vi "test Buffer String to Display String.vi"(8 "error in (no error)":errorcluster, 11 "TestCase in":refnum<class "Buffer Tests.lvclass">=refnum) -> (0 "error out":errorcluster, 3 "TestCase out":refnum<class "Buffer Tests.lvclass">)   [LabVIEW 2021, in "Buffer Tests.lvclass"]
uses:
  Buffer Tests.lvclass
  DSF Core.lvlib
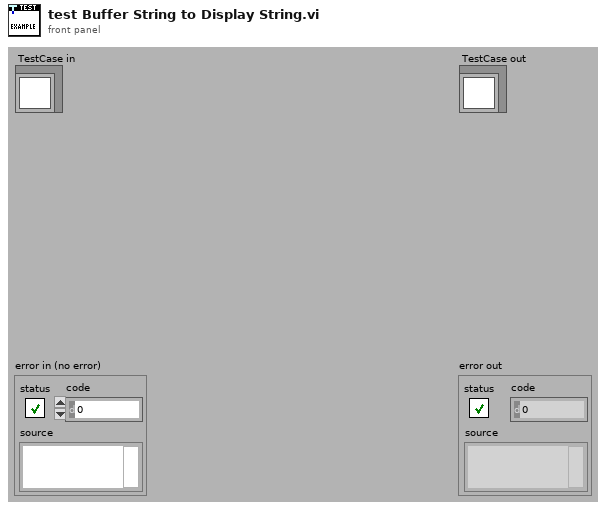
[diagram p1: front panel]
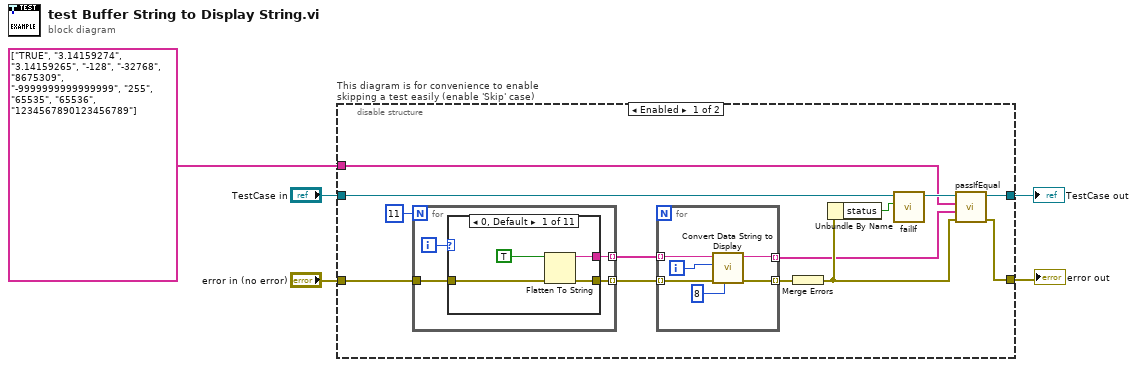
[diagram p0: block diagram]
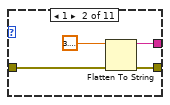
[diagram p2: hidden frame]
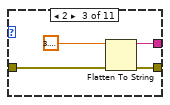
[diagram p3: hidden frame]
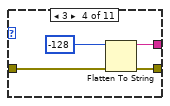
[diagram p4: hidden frame]
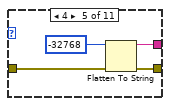
[diagram p5: hidden frame]
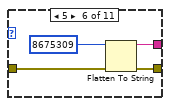
[diagram p6: hidden frame]
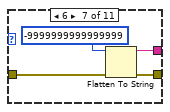
[diagram p7: hidden frame]
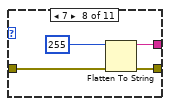
[diagram p8: hidden frame]
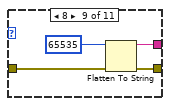
[diagram p9: hidden frame]
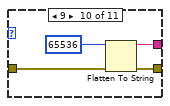
[diagram p10: hidden frame]
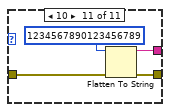
[diagram p11: hidden frame]
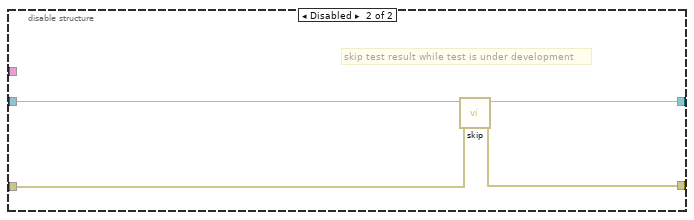
[diagram p12: hidden frame]
diagram:
  n1 = disable-structure "This diagram is for convenience to enable skipping a test easily (enable 'Skip' case)" shown="Enabled" {
    disable-tunnel: "TestCase in" -> [w12 w76]
    disable-tunnel: [w18 w74] -> w2
    disable-tunnel: [w17 w75] -> w4
    disable-tunnel: "error in (no error)" -> [w16 w73]
    disable-tunnel: string[] ["TRUE", "3.14159274", "3.14159265", "-128", "-32768", "8675309", "-9999999999999999", "255", "65535", "65536", "1234567890123456789"] ("Array") -> [w7 _]
    frame Enabled {
      n2 = for {
        N: 11 -> [_]
        tunnel: [w27] -> w15 mode=indexing
        tunnel: w16 -> [w26]
        tunnel: [w25] -> w14 mode=indexing
        i -> [w28]
        n3 = case shown="0, Default" w28 {
          tunnel: [w31 w35 w39 w43 w47 w51 w55 w59 w63 w67 w71] -> w27
          tunnel: w26 -> [w30 w34 w38 w42 w46 w50 w54 w58 w62 w66 w70]
          tunnel: [w29 w33 w37 w41 w45 w49 w53 w57 w61 w65 w69] -> w25
          frame 0, Default {
            n4 = Flatten To String(anything=TRUE, error in (no error)=w30) -> (data string=w31:string, error out=w29:errorcluster)  [unwired: 2 in, 1 out]
          }
          frame 1 {
            n5 = Flatten To String(anything=sgl 3.1415927, error in (no error)=w34) -> (data string=w35:string, error out=w33:errorcluster)  [unwired: 2 in, 1 out]
          }
          frame 2 {
            n6 = Flatten To String(anything=3.141592653589793, error in (no error)=w38) -> (data string=w39:string, error out=w37:errorcluster)  [unwired: 2 in, 1 out]
          }
          frame 3 {
            n7 = Flatten To String(anything=i8 -128, error in (no error)=w42) -> (data string=w43:string, error out=w41:errorcluster)  [unwired: 2 in, 1 out]
          }
          frame 4 {
            n8 = Flatten To String(anything=i16 -32768, error in (no error)=w46) -> (data string=w47:string, error out=w45:errorcluster)  [unwired: 2 in, 1 out]
          }
          frame 5 {
            n9 = Flatten To String(anything=8675309, error in (no error)=w50) -> (data string=w51:string, error out=w49:errorcluster)  [unwired: 2 in, 1 out]
          }
          frame 6 {
            n10 = Flatten To String(anything=i64 -9999999999999999, error in (no error)=w54) -> (data string=w55:string, error out=w53:errorcluster)  [unwired: 2 in, 1 out]
          }
          frame 7 {
            n11 = Flatten To String(anything=u8 255, error in (no error)=w58) -> (data string=w59:string, error out=w57:errorcluster)  [unwired: 2 in, 1 out]
          }
          frame 8 {
            n12 = Flatten To String(anything=u16 65535, error in (no error)=w62) -> (data string=w63:string, error out=w61:errorcluster)  [unwired: 2 in, 1 out]
          }
          frame 9 {
            n13 = Flatten To String(anything=u32 65536, error in (no error)=w66) -> (data string=w67:string, error out=w65:errorcluster)  [unwired: 2 in, 1 out]
          }
          frame 10 {
            n14 = Flatten To String(anything=u64 1234567890123456789, error in (no error)=w70) -> (data string=w71:string, error out=w69:errorcluster)  [unwired: 2 in, 1 out]
          }
        }
      }
      n15 = for {
        tunnel: w15 -> [w24] mode=indexing
        tunnel: w14 -> [w23] mode=indexing
        tunnel: [w21] -> w6 mode=indexing
        tunnel: [w20] -> w13 mode=indexing
        i -> [w22]
        n16 = call "Convert Data String to Display.vi"("precision (3)"=i16 8, "error in"=w23, "string data type"=w22, "data string"=w24) -> ("error out"=w20:errorcluster, "display string"=w21:string)  [unwired: 6 in]
      }
      n17 = Merge Errors(w13) -> (w10:errorcluster)
      n18 = Unbundle By Name(w10) -> ("status"=w9:bool)
      n19 = call-dynamic "failIf.vi"("fail"=w9, "TestCase in"=w12) -> ("TestCase out"=w11:refnum<class "Buffer Tests.lvclass">)  [unwired: 8 in, 1 out]
      n20 = call-dynamic "passIfEqual.vi"("error in (no error)"=w10, "y"=w6, "x"=w7, "TestCase in"=w11) -> ("error out"=w17:errorcluster, "TestCase out"=w18:refnum<class "Buffer Tests.lvclass">)  [unwired: 6 in]
    }
    frame Disabled {
      # "skip test result while test is under development"
      n21 = call <vilib>:"skip.vi"("error in (no error)"=w73, "TestCase in"=w76) -> ("error out"=w75:errorcluster, "TestCase out"=w74:refnum<class "Buffer Tests.lvclass">)  [unwired: 8 in]
    }
  }
  "error out" <- w4
  "TestCase out" <- w2
